vi "Analog Replays Page Wrapper.vi"(8 "error in (no error)":errorcluster, 11 "Node Ptr":T1 format="%.0x") -> (0 "error out":errorcluster)   [LabVIEW 2015, in "Engine Simulation Toolkit System Explorer.lvlib"]
uses:
  Engine Simulation Toolkit System Explorer.lvlib
  <vilib>/NI Veristand/Custom Device API/Custom Device Item Ref.ctl
  Analog Replays Page - Multi FPGA.vi
  Analog Replays Page.vi
  Shared/Constants and GUIDs.vi
  Shared/Engine Simulation Toolkit Shared.lvlib
  <vilib>/NI Veristand/Custom Device API/Custom Device API.lvlib
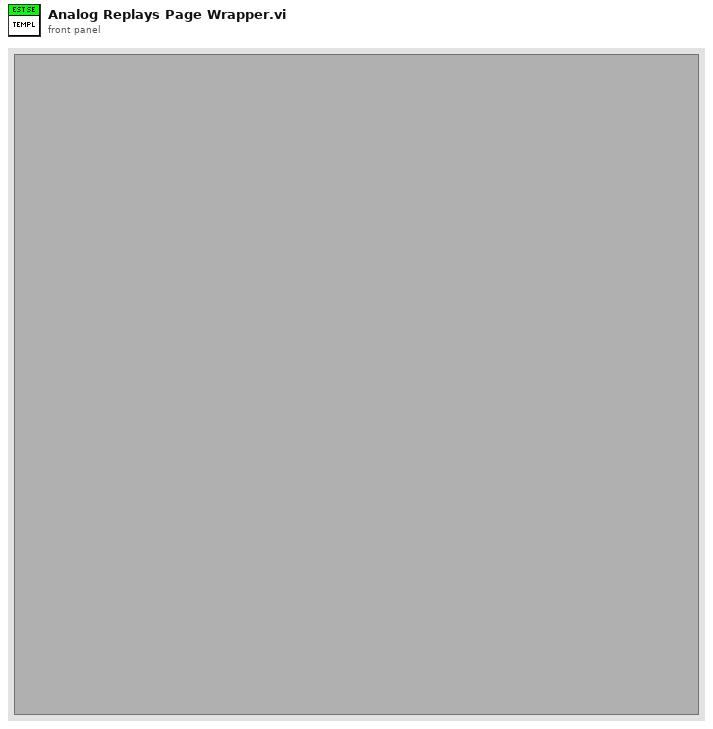
[diagram p1: front panel]
types:
  T1 = typedef "Custom Device API.lvlib/Custom Device Item Ref.ctl" = u64
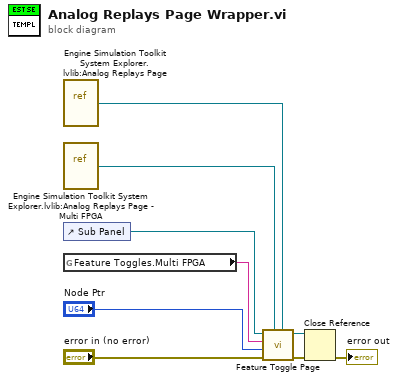
[diagram p0: block diagram]
diagram:
  n1 = vi-ref "Engine Simulation Toolkit System Explorer.lvlib:Analog Replays Page.vi"() -> (w6:refnum<vi>)
  n2 = vi-ref "Engine Simulation Toolkit System Explorer.lvlib:Analog Replays Page - Multi FPGA.vi"() -> (w5:refnum<vi>)
  n3 = control-ref of="Sub Panel"() -> (w7:refnum<vi>)
  n4 = global read "Constants and GUIDs.vi" "Feature Toggles.Multi FPGA"() -> (w4:string)
  n5 = call "Feature Toggle Page.vi"("feature disabled vi"=w6, "feature enabled vi"=w5, "error in (no error)"="error in (no error)", "Node Ptr"="Node Ptr", "feature name"=w4, "SubPanel in"=w7) -> ("error out"=w2:errorcluster, "SubPanel out"=w1:refnum<vi>)  [unwired: 4 in]
  n6 = Close Reference(reference=w1, error in (no error)=w2) -> (error out=→"error out":errorcluster)
